vi "Traction Receipe Run Trial.vi"() -> ()   [LabVIEW 2025]
uses:
  Traction Receipe Enum.ctl
panel:
  out "SET entrainment Velocity":dbl
  out "Test Array Size":i32
  in  "SRR INDEX [ STRIBECK]":i32
  out "Stribeck Size":i32
  out "SET SRR":dbl
  out "Enum - READ":T1
  out "ELAPSED TIMER":dbl
  in  "START":bool
  out "BALL SET RPM":dbl
  out "DISC SET RPM":dbl
  in  "LOAD READ":dbl
  out "SET LOAD":dbl
  in  "TEMPERATURE READ":dbl
  out "SET TEMPERATURE":dbl
  out "Traction Size":i32
  out "DISC SPEED (rpm)":dbl=100.0 min=0.1 max=3000.0 step=0.1 format="%.1f"
  out "BALL SPEED (rpm)":dbl=100.0 min=0.1 max=3000.0 step=0.1 format="%.1f"
  in  "BALL WEAR TRACK":dbl=7.9
  in  "DISC WEARTRACK":dbl=16.0
  in  "SRR INDEX [ TRACTION]":i32
  in  "Start Index Type":i32
  in  "Enum - Menu":T1
  out "Ball (mm/sec)":dbl
  out "Disc (mm/sec)":dbl
  in  "Multicolumn Listbox":i32(listbox)
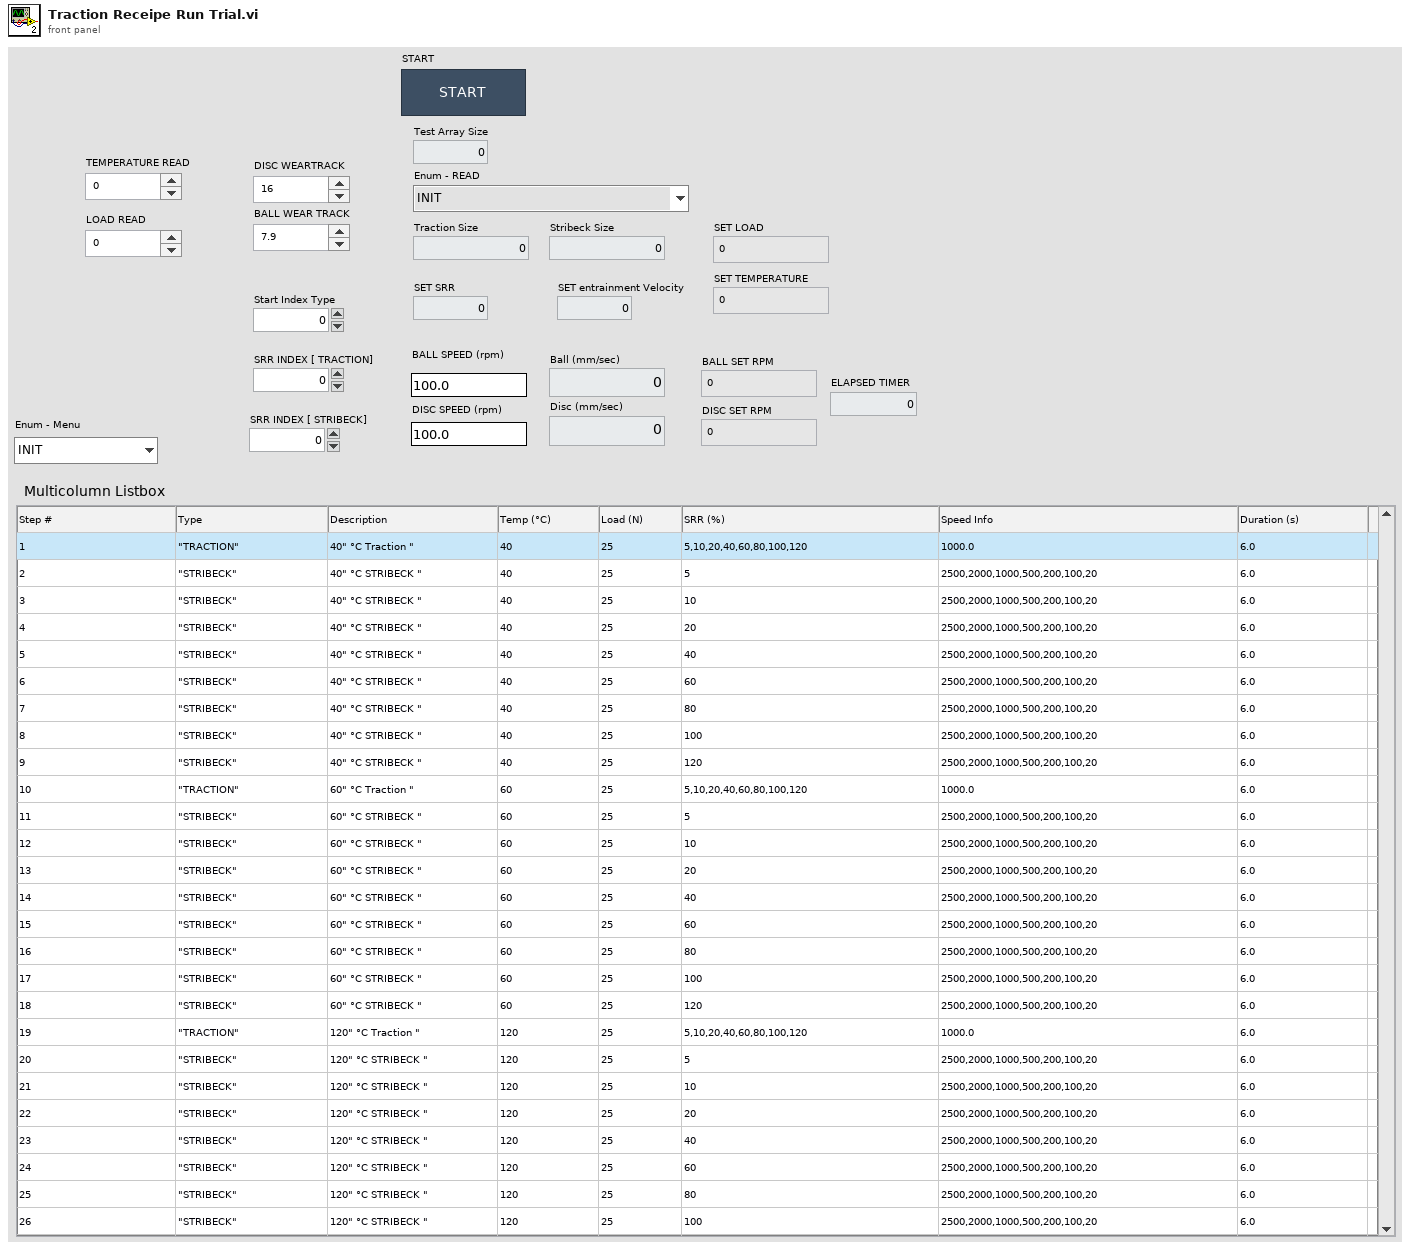
[diagram p1: front panel]
types:
  T1 = typedef "Traction Receipe Enum.ctl" = enum16{"INIT", "START", "TRACTION", "STRIBECK", "MAIN INDEX INCREMENT", "TEMPERATURE SET", "TEMPERATURE REACH", "CHURNING START", "CHURNING STOP", "LOAD", "LOAD REACHED", "SRR SET", "SRR WAIT", "SRR INCREMENT", "SPEED SET", "SPEED WAIT", "SPEED INCREMENT", "UNLOAD", "CLOSE"}
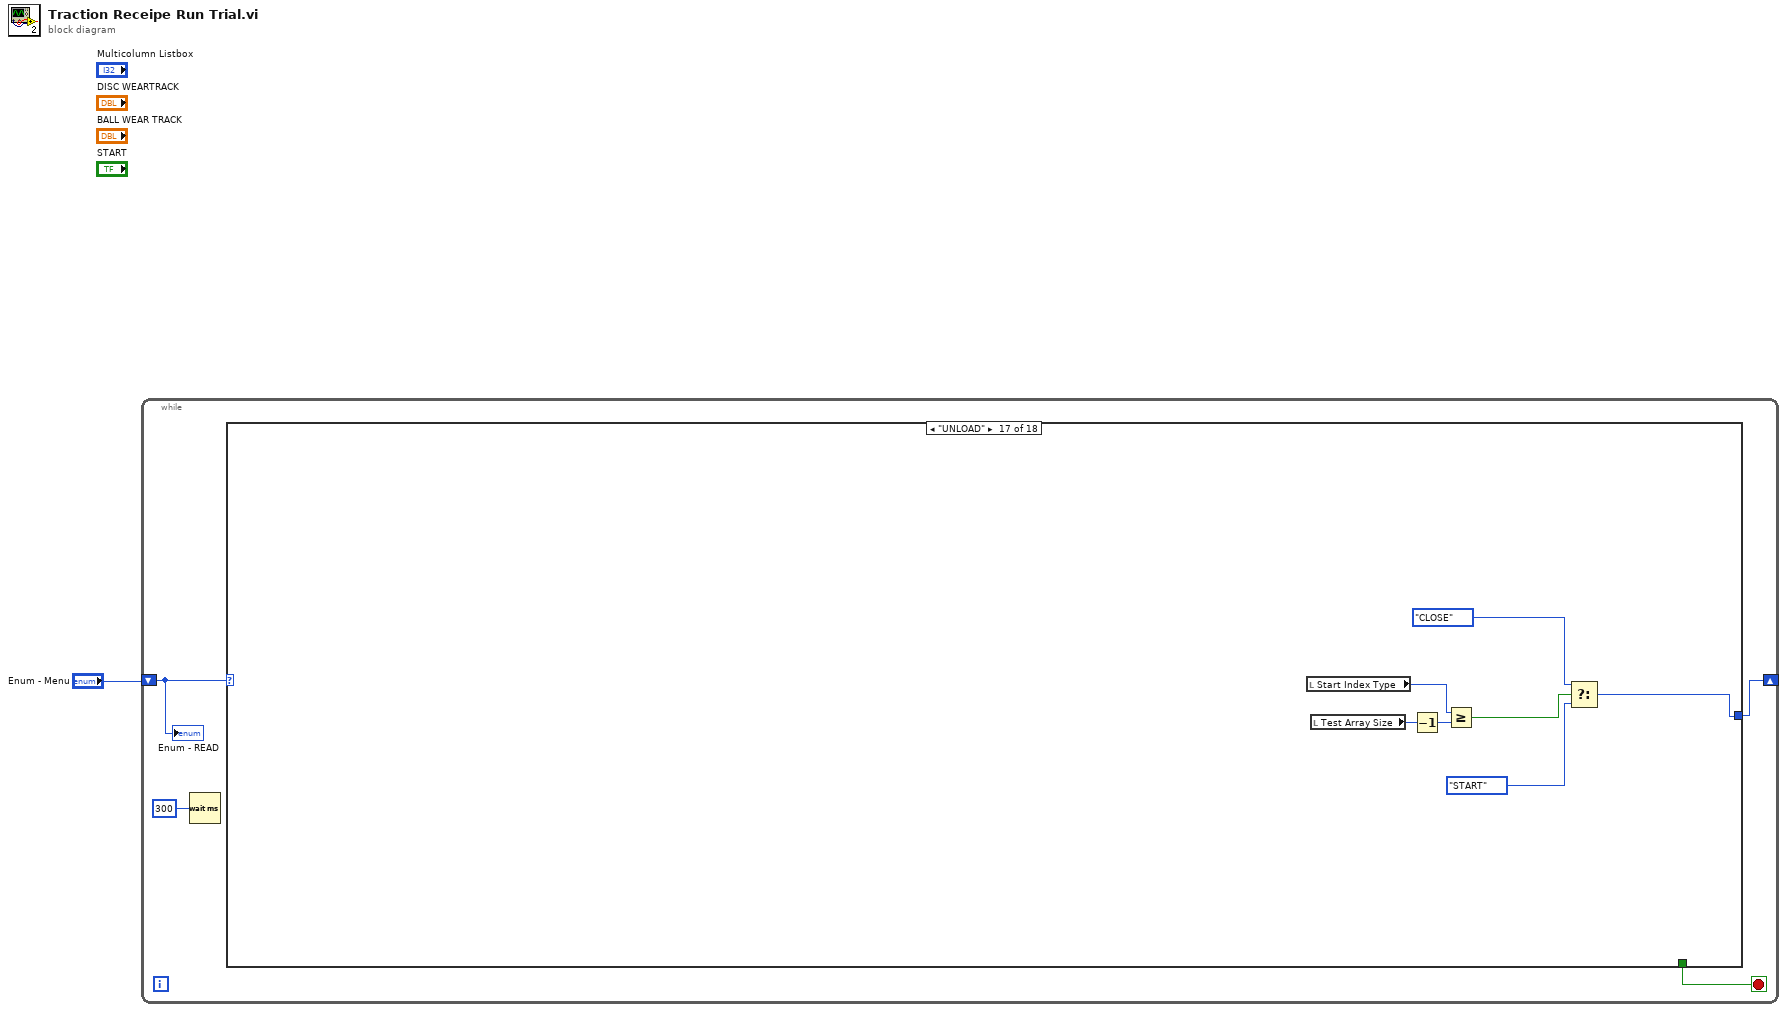
[diagram p0: block diagram]
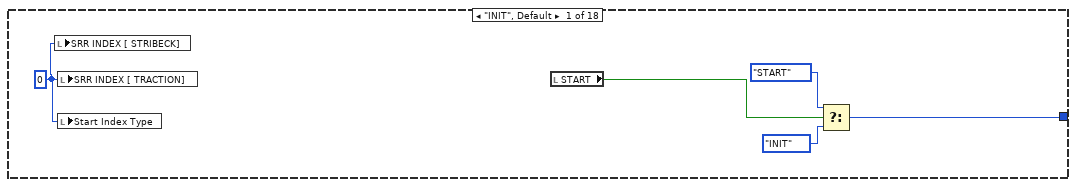
[diagram p2: hidden frame]
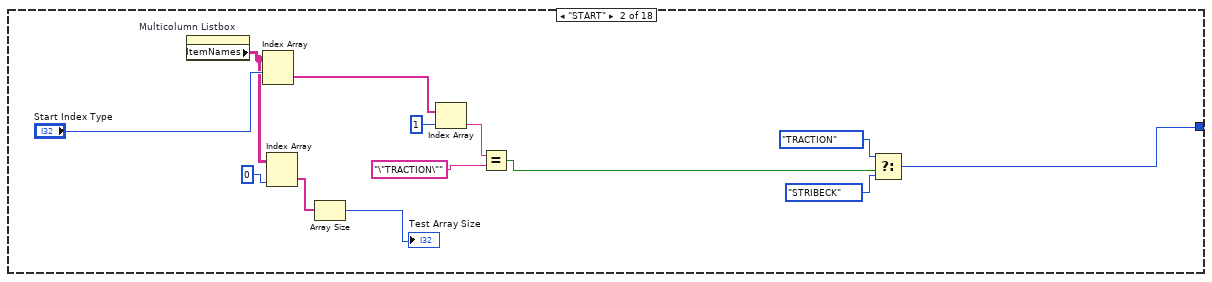
[diagram p3: hidden frame]
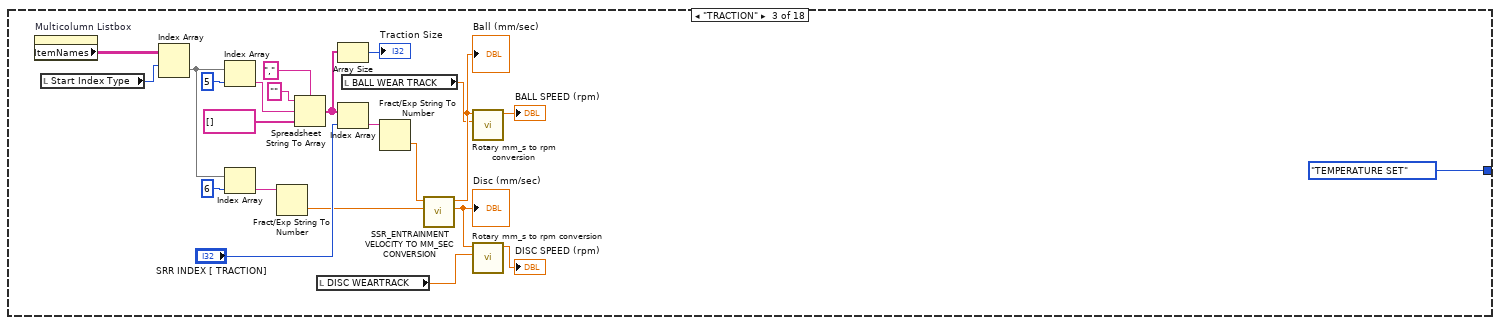
[diagram p4: hidden frame]
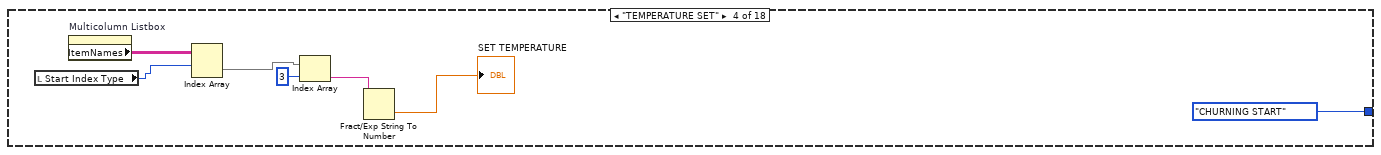
[diagram p5: hidden frame]
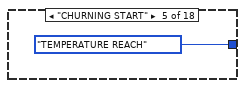
[diagram p6: hidden frame]
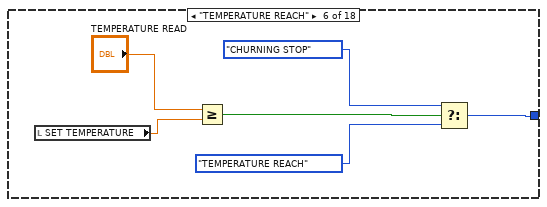
[diagram p7: hidden frame]
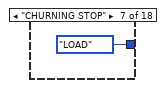
[diagram p8: hidden frame]
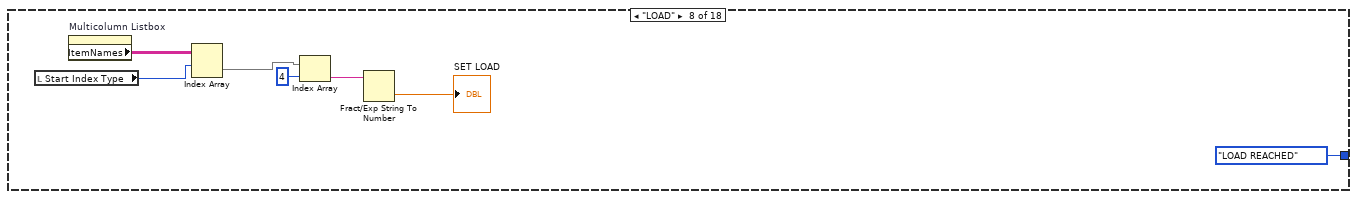
[diagram p9: hidden frame]
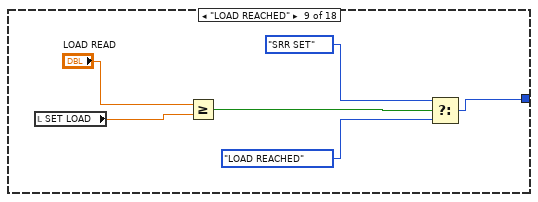
[diagram p10: hidden frame]
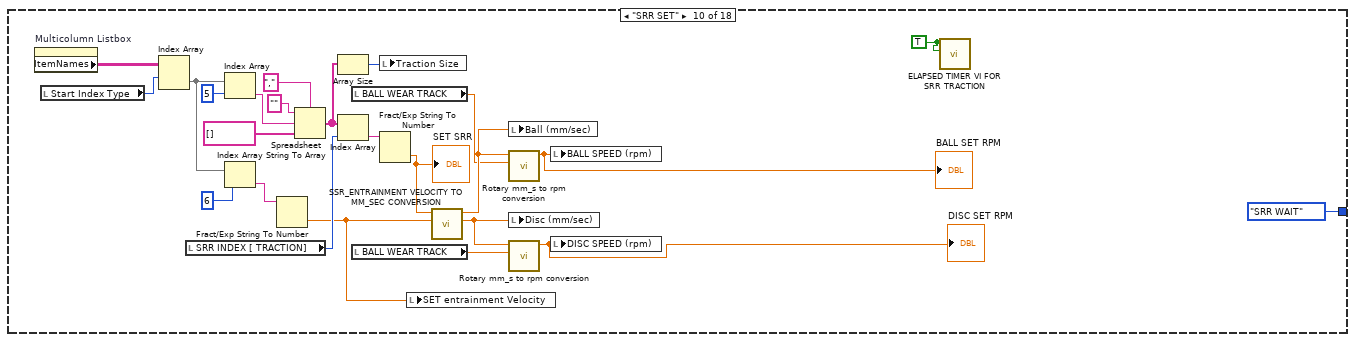
[diagram p11: hidden frame]
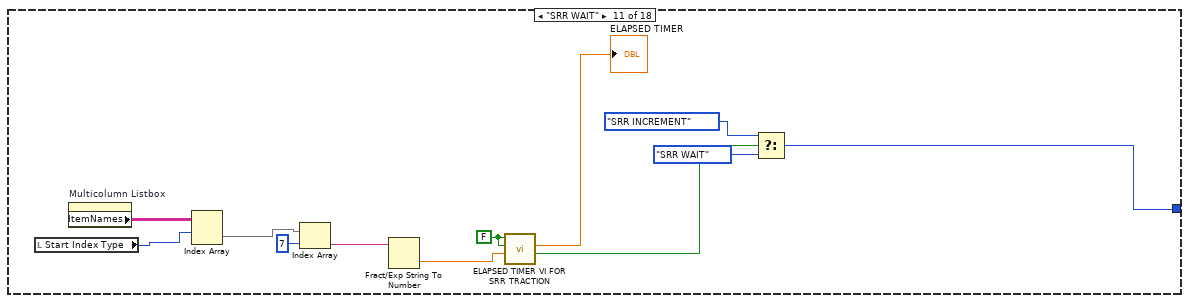
[diagram p12: hidden frame]
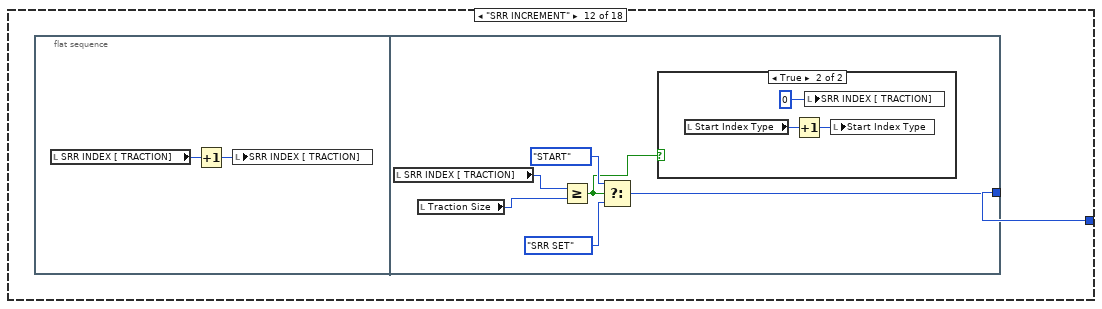
[diagram p13: hidden frame]
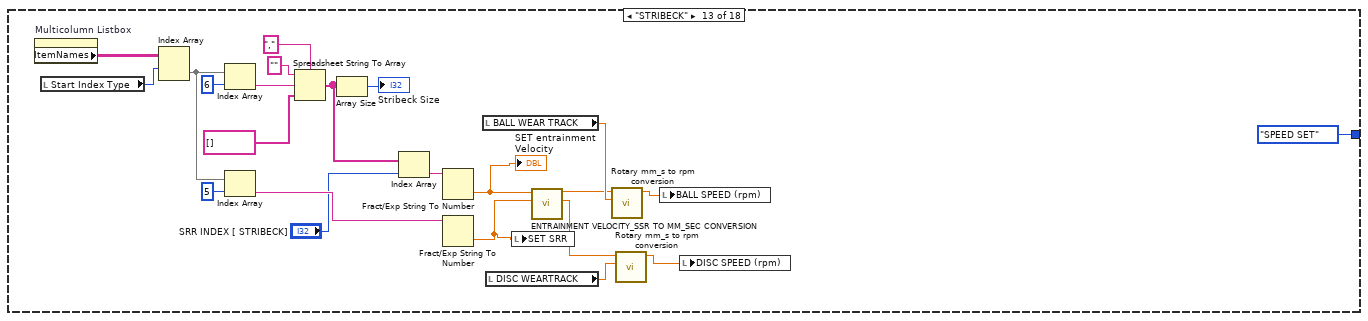
[diagram p15: hidden frame]
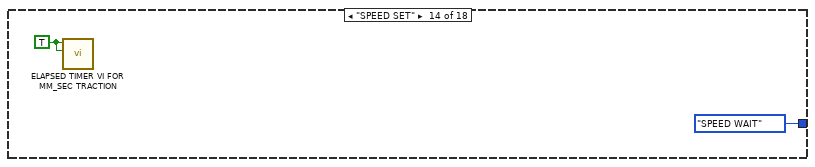
[diagram p16: hidden frame]
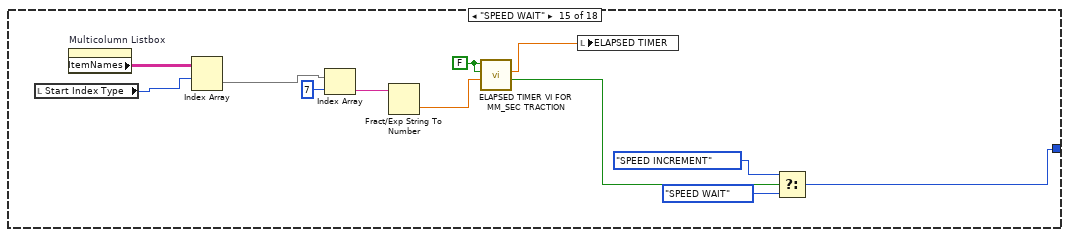
[diagram p17: hidden frame]
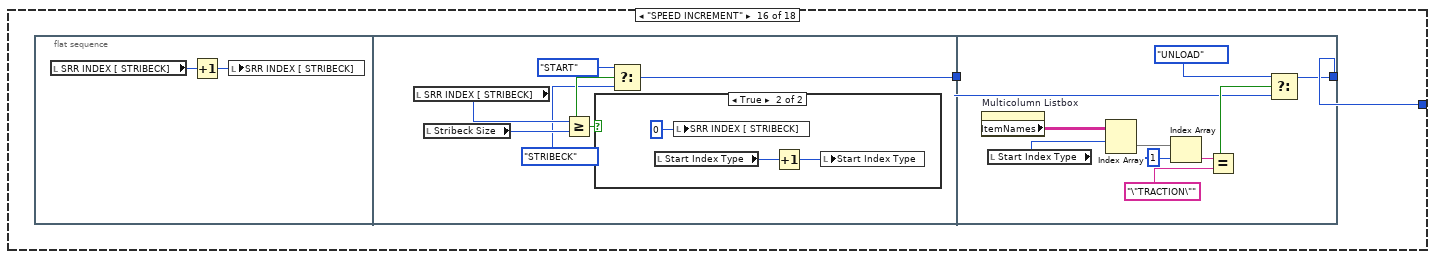
[diagram p18: hidden frame]
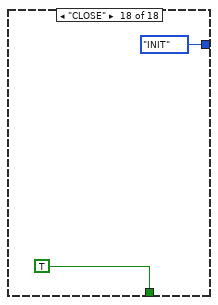
[diagram p20: hidden frame]
diagram:
  n1 = while {
    shift-right: [w4] -> _
    shift-left: "Enum - Menu" -> [w5]
    stop <- w3 stop-if-true
    n2 = Wait (ms)(milliseconds to wait=u32 300) -> ()  [unwired: 1 out]
    n3 = case shown="\"UNLOAD\"" w5 {
      tunnel: [w8 w15 Traction_Receipe_Enum."TEMPERATURE SET" ("Enum - Menu") Traction_Receipe_Enum."CHURNING START" ("Enum - Menu") Traction_Receipe_Enum."TEMPERATURE REACH" ("Enum - Menu") w55 Traction_Receipe_Enum."LOAD" ("Enum - Menu") Traction_Receipe_Enum."LOAD REACHED" ("Enum - Menu") w71 Traction_Receipe_Enum."SRR WAIT" ("Enum - Menu") w101 w111 Traction_Receipe_Enum."SPEED SET" ("Enum - Menu") Traction_Receipe_Enum."SPEED WAIT" ("Enum - Menu") w148 w161 w184 Traction_Receipe_Enum."INIT" ("Enum - Menu")] -> w4
      tunnel: [_ _ _ _ _ _ _ _ _ _ _ _ _ _ _ _ _ TRUE] -> w3
      frame "INIT", Default {
        w6 = 0 ("Start Index")
        n4 = local write "SRR INDEX [ STRIBECK]"(w6) -> ()
        n5 = local write "SRR INDEX [ TRACTION]"(w6) -> ()
        n6 = local write "Start Index Type"(w6) -> ()
        n7 = local read "START"() -> (w7:bool)
        n8 = Select(t=Traction_Receipe_Enum."START" ("Enum - Menu"), s=w7, f=Traction_Receipe_Enum."INIT" ("Enum - Menu")) -> (s? t:f=w8:T1)
      }
      frame "START" {
        n9 = property on="Multicolumn Listbox" class="MCListbox (strict)"() -> ("ItemNames"=w14:string[][])  [unwired: 2 in, 2 out]
        n10 = Index Array(array=w14, index (row)="Start Index Type") -> (element=w19:string[])  [unwired: 1 in]
        n11 = Index Array(array=w14, index (col)=0 ("index (row)")) -> (element=w13:string[])  [unwired: 1 in]
        n12 = Array Size(array=w13) -> (size(s)=→"Test Array Size":i32)
        n13 = Index Array(array=w19, index=1) -> (element=w21:string)
        n14 = Equal?(x=w21, y="\"TRACTION\"") -> (x = y?=w16:bool)
        n15 = Select(t=Traction_Receipe_Enum."TRACTION" ("Enum - Menu"), s=w16, f=Traction_Receipe_Enum."STRIBECK" ("Enum - Menu")) -> (s? t:f=w15:T1)
      }
      frame "TRACTION" {
        n16 = property on="Multicolumn Listbox" class="MCListbox (strict)"() -> ("ItemNames"=w41:string[][])  [unwired: 2 in, 2 out]
        n17 = local read "Start Index Type"() -> (w25:i32)
        n18 = Index Array(array=w41, index (row)=w25) -> (element=w40:string[])  [unwired: 1 in]
        n19 = Index Array(array=w40, index=5) -> (element=w39:string)
        n20 = Index Array(array=w40, index=6) -> (element=w34:string)
        n21 = Fract/Exp String To Number(string=w34) -> (number=w37:dbl)  [unwired: 3 in, 1 out]
        n22 = Spreadsheet String To Array(delimiter (Tab)=",", format string="", spreadsheet string=w39, array type (2D Dbl)=string[] []) -> (array=w28:string[])
        n23 = local read "DISC WEARTRACK"() -> (w24:dbl)
        n24 = Array Size(array=w28) -> (size(s)=→"Traction Size":i32)
        n25 = Index Array(array=w28, index="SRR INDEX [ TRACTION]") -> (element=w35:string)
        n26 = local read "BALL WEAR TRACK"() -> (w32:dbl)
        n27 = Fract/Exp String To Number(string=w35) -> (number=w36:dbl)  [unwired: 3 in, 1 out]
        n28 = call "SSR_ENTRAINMENT VELOCITY TO MM_SEC CONVERSION.vi"("Entrainment Speed"=w37, "Initial SSR"=w36) -> ("Disc"=w31:dbl, "Ball"=w33:dbl)  [unwired: 7 in, 1 out]
        "Disc (mm/sec)" <- w31
        "Ball (mm/sec)" <- w33
        n29 = call "Rotary mm_s to rpm conversion.vi"("Wear Track Diameter"=w32, "Enter initial Velocity (m/s)  3"=w33) -> ("Initial Speed (RPM) 2"=→"BALL SPEED (rpm)":dbl)  [unwired: 7 in, 2 out]
        n30 = call "Rotary mm_s to rpm conversion.vi"("Wear Track Diameter"=w24, "Enter initial Velocity (m/s)  3"=w31) -> ("Initial Speed (RPM) 2"=→"DISC SPEED (rpm)":dbl)  [unwired: 7 in, 2 out]
      }
      frame "TEMPERATURE SET" {
        n31 = local read "Start Index Type"() -> (w47:i32)
        n32 = property on="Multicolumn Listbox" class="MCListbox (strict)"() -> ("ItemNames"=w51:string[][])  [unwired: 2 in, 2 out]
        n33 = Index Array(array=w51, index (row)=w47) -> (element=w52:string[])  [unwired: 1 in]
        n34 = Index Array(array=w52, index=3) -> (element=w49:string)
        n35 = Fract/Exp String To Number(string=w49) -> (number=→"SET TEMPERATURE":dbl)  [unwired: 3 in, 1 out]
      }
      frame "CHURNING START" {
      }
      frame "TEMPERATURE REACH" {
        n36 = local read "SET TEMPERATURE"() -> (w59:dbl)
        n37 = Greater Or Equal?(x="TEMPERATURE READ", y=w59) -> (x >= y?=w58:bool)
        n38 = Select(t=Traction_Receipe_Enum."CHURNING STOP" ("Enum - Menu"), s=w58, f=Traction_Receipe_Enum."TEMPERATURE REACH" ("Enum - Menu")) -> (s? t:f=w55:T1)
      }
      frame "CHURNING STOP" {
      }
      frame "LOAD" {
        n39 = local read "Start Index Type"() -> (w62:i32)
        n40 = property on="Multicolumn Listbox" class="MCListbox (strict)"() -> ("ItemNames"=w67:string[][])  [unwired: 2 in, 2 out]
        n41 = Index Array(array=w67, index (row)=w62) -> (element=w68:string[])  [unwired: 1 in]
        n42 = Index Array(array=w68, index=4) -> (element=w66:string)
        n43 = Fract/Exp String To Number(string=w66) -> (number=→"SET LOAD":dbl)  [unwired: 3 in, 1 out]
      }
      frame "LOAD REACHED" {
        n44 = local read "SET LOAD"() -> (w69:dbl)
        n45 = Greater Or Equal?(x="LOAD READ", y=w69) -> (x >= y?=w74:bool)
        n46 = Select(t=Traction_Receipe_Enum."SRR SET" ("Enum - Menu"), s=w74, f=Traction_Receipe_Enum."LOAD REACHED" ("Enum - Menu")) -> (s? t:f=w71:T1)
      }
      frame "SRR SET" {
        w97 = TRUE ("PAUSE")
        n47 = property on="Multicolumn Listbox" class="MCListbox (strict)"() -> ("ItemNames"=w92:string[][])  [unwired: 2 in, 2 out]
        n48 = local read "Start Index Type"() -> (w83:i32)
        n49 = Index Array(array=w92, index (row)=w83) -> (element=w91:string[])  [unwired: 1 in]
        n50 = local read "SRR INDEX [ TRACTION]"() -> (w95:i32)
        n51 = Index Array(array=w91, index=5) -> (element=w90:string)
        n52 = Index Array(array=w91, index=6) -> (element=w87:string)
        n53 = Fract/Exp String To Number(string=w87) -> (number=w75:dbl)  [unwired: 3 in, 1 out]
        n54 = Spreadsheet String To Array(delimiter (Tab)=",", format string="", spreadsheet string=w90, array type (2D Dbl)=string[] []) -> (array=w84:string[])
        n55 = Array Size(array=w84) -> (size(s)=w96:i32)
        n56 = Index Array(array=w84, index=w95) -> (element=w88:string)
        n57 = local read "BALL WEAR TRACK"() -> (w86:dbl)
        n58 = local read "BALL WEAR TRACK"() -> (w85:dbl)
        n59 = local write "Traction Size"(w96) -> ()
        n60 = Fract/Exp String To Number(string=w88) -> (number=w89:dbl)  [unwired: 3 in, 1 out]
        "SET SRR" <- w89
        n61 = local write "SET entrainment Velocity"(w75) -> ()
        n62 = call "SSR_ENTRAINMENT VELOCITY TO MM_SEC CONVERSION.vi"("Entrainment Speed"=w75, "Initial SSR"=w89) -> ("Disc"=w94:dbl, "Ball"=w93:dbl)  [unwired: 7 in, 1 out]
        n63 = local write "Ball (mm/sec)"(w93) -> ()
        n64 = call "Rotary mm_s to rpm conversion.vi"("Wear Track Diameter"=w86, "Enter initial Velocity (m/s)  3"=w93) -> ("Initial Speed (RPM) 2"=w77:dbl)  [unwired: 7 in, 2 out]
        "BALL SET RPM" <- w77
        n65 = local write "Disc (mm/sec)"(w94) -> ()
        n66 = call "Rotary mm_s to rpm conversion.vi"("Wear Track Diameter"=w85, "Enter initial Velocity (m/s)  3"=w94) -> ("Initial Speed (RPM) 2"=w76:dbl)  [unwired: 7 in, 2 out]
        "DISC SET RPM" <- w76
        n67 = local write "BALL SPEED (rpm)"(w77) -> ()
        n68 = local write "DISC SPEED (rpm)"(w76) -> ()
        n69 = call "ELAPSED TIMER VI FOR SRR TRACTION.vi"("RESET"=w97, "PAUSE"=w97) -> ()  [unwired: 7 in, 3 out]
      }
      frame "SRR WAIT" {
        w106 = FALSE ("PAUSE")
        n70 = local read "Start Index Type"() -> (w99:i32)
        n71 = property on="Multicolumn Listbox" class="MCListbox (strict)"() -> ("ItemNames"=w109:string[][])  [unwired: 2 in, 2 out]
        n72 = Index Array(array=w109, index (row)=w99) -> (element=w110:string[])  [unwired: 1 in]
        n73 = Index Array(array=w110, index=7) -> (element=w108:string)
        n74 = Fract/Exp String To Number(string=w108) -> (number=w105:dbl)  [unwired: 3 in, 1 out]
        n75 = call "ELAPSED TIMER VI FOR SRR TRACTION.vi"("TARGET"=w105, "RESET"=w106, "PAUSE"=w106) -> ("ELAPSED INDICATION"=w104:bool, "ELAPSED TIMER"=→"ELAPSED TIMER":dbl)  [unwired: 6 in, 1 out]
        n76 = Select(t=Traction_Receipe_Enum."SRR INCREMENT" ("Enum - Menu"), s=w104, f=Traction_Receipe_Enum."SRR WAIT") -> (s? t:f=w101:T1)
      }
      frame "SRR INCREMENT" {
        n77 = flat-sequence {
          tunnel: [w116] -> w111
          frame #0 {
            n78 = local read "SRR INDEX [ TRACTION]"() -> (w113:i32)
            n79 = Increment(x=w113) -> (x+1=w112:i32)
            n80 = local write "SRR INDEX [ TRACTION]"(w112) -> ()
          }
          frame #1 {
            n81 = local read "SRR INDEX [ TRACTION]"() -> (w114:i32)
            n82 = local read "Traction Size"() -> (w119:i32)
            n83 = Greater Or Equal?(x=w114, y=w119) -> (x >= y?=w115:bool)
            n84 = Select(t=Traction_Receipe_Enum."START" ("Enum - Menu"), s=w115, f=Traction_Receipe_Enum."SRR SET" ("Enum - Menu")) -> (s? t:f=w116:T1)
            n85 = case shown="True" w115 {
              frame False {
              }
              frame True {
                n86 = local read "Start Index Type"() -> (w122:i32)
                n87 = Increment(x=w122) -> (x+1=w121:i32)
                n88 = local write "SRR INDEX [ TRACTION]"(0 ("SRR INDEX [ TRACTION]")) -> ()
                n89 = local write "Start Index Type"(w121) -> ()
              }
            }
          }
        }
      }
      frame "STRIBECK" {
        n90 = property on="Multicolumn Listbox" class="MCListbox (strict)"() -> ("ItemNames"=w130:string[][])  [unwired: 2 in, 2 out]
        n91 = local read "Start Index Type"() -> (w131:i32)
        n92 = Index Array(array=w130, index (row)=w131) -> (element=w134:string[])  [unwired: 1 in]
        n93 = Index Array(array=w134, index=6) -> (element=w132:string)
        n94 = Index Array(array=w134, index=5) -> (element=w138:string)
        n95 = Spreadsheet String To Array(delimiter (Tab)=",", format string="", spreadsheet string=w132, array type (2D Dbl)=string[] []) -> (array=w136:string[])
        n96 = Array Size(array=w136) -> (size(s)=→"Stribeck Size":i32)
        n97 = Index Array(array=w136, index="SRR INDEX [ STRIBECK]") -> (element=w137:string)
        n98 = Fract/Exp String To Number(string=w137) -> (number=w124:dbl)  [unwired: 3 in, 1 out]
        "SET entrainment Velocity" <- w124
        n99 = Fract/Exp String To Number(string=w138) -> (number=w123:dbl)  [unwired: 3 in, 1 out]
        n100 = local read "BALL WEAR TRACK"() -> (w140:dbl)
        n101 = local read "DISC WEARTRACK"() -> (w142:dbl)
        n102 = local write "SET SRR"(w123) -> ()
        n103 = call "ENTRAINMENT VELOCITY_SSR TO MM_SEC CONVERSION.vi"("SSR"=w123, "INITIAL Entrainment Speed"=w124) -> ("Disc"=w141:dbl, "Ball"=w139:dbl)  [unwired: 7 in, 1 out]
        n104 = call "Rotary mm_s to rpm conversion.vi"("Wear Track Diameter"=w140, "Enter initial Velocity (m/s)  3"=w139) -> ("Initial Speed (RPM) 2"=w143:dbl)  [unwired: 7 in, 2 out]
        n105 = call "Rotary mm_s to rpm conversion.vi"("Wear Track Diameter"=w142, "Enter initial Velocity (m/s)  3"=w141) -> ("Initial Speed (RPM) 2"=w144:dbl)  [unwired: 7 in, 2 out]
        n106 = local write "BALL SPEED (rpm)"(w143) -> ()
        n107 = local write "DISC SPEED (rpm)"(w144) -> ()
      }
      frame "SPEED SET" {
        w146 = TRUE ("PAUSE")
        n108 = call "ELAPSED TIMER VI FOR MM_SEC TRACTION.vi"("RESET"=w146, "PAUSE"=w146) -> ()  [unwired: 7 in, 3 out]
      }
      frame "SPEED WAIT" {
        w153 = FALSE ("PAUSE")
        n109 = local read "Start Index Type"() -> (w156:i32)
        n110 = property on="Multicolumn Listbox" class="MCListbox (strict)"() -> ("ItemNames"=w158:string[][])  [unwired: 2 in, 2 out]
        n111 = Index Array(array=w158, index (row)=w156) -> (element=w159:string[])  [unwired: 1 in]
        n112 = Index Array(array=w159, index=7) -> (element=w157:string)
        n113 = Fract/Exp String To Number(string=w157) -> (number=w154:dbl)  [unwired: 3 in, 1 out]
        n114 = call "ELAPSED TIMER VI FOR MM_SEC TRACTION.vi"("TARGET"=w154, "RESET"=w153, "PAUSE"=w153) -> ("ELAPSED INDICATION"=w149:bool, "ELAPSED TIMER"=w152:dbl)  [unwired: 6 in, 1 out]
        n115 = local write "ELAPSED TIMER"(w152) -> ()
        n116 = Select(t=Traction_Receipe_Enum."SPEED INCREMENT" ("Enum - Menu"), s=w149, f=Traction_Receipe_Enum."SPEED WAIT") -> (s? t:f=w148:T1)
      }
      frame "SPEED INCREMENT" {
        n117 = flat-sequence {
          tunnel: [w164] -> w160
          tunnel: [w176] -> w161
          tunnel: w160 -> [w174]
          frame #0 {
            n118 = local read "SRR INDEX [ STRIBECK]"() -> (w163:i32)
            n119 = Increment(x=w163) -> (x+1=w162:i32)
            n120 = local write "SRR INDEX [ STRIBECK]"(w162) -> ()
          }
          frame #1 {
            n121 = local read "SRR INDEX [ STRIBECK]"() -> (w168:i32)
            n122 = local read "Stribeck Size"() -> (w169:i32)
            n123 = Greater Or Equal?(x=w168, y=w169) -> (x >= y?=w166:bool)
            n124 = case shown="True" w166 {
              frame False {
              }
              frame True {
                n125 = local read "Start Index Type"() -> (w172:i32)
                n126 = local write "SRR INDEX [ STRIBECK]"(0 ("SRR INDEX [ STRIBECK]")) -> ()
                n127 = Increment(x=w172) -> (x+1=w171:i32)
                n128 = local write "Start Index Type"(w171) -> ()
              }
            }
            n129 = Select(t=Traction_Receipe_Enum."START" ("Enum - Menu"), s=w166, f=Traction_Receipe_Enum."STRIBECK") -> (s? t:f=w164:T1)
          }
          frame #2 {
            n130 = property on="Multicolumn Listbox" class="MCListbox (strict)"() -> ("ItemNames"=w181:string[][])  [unwired: 2 in, 2 out]
            n131 = local read "Start Index Type"() -> (w182:i32)
            n132 = Index Array(array=w181, index (row)=w182) -> (element=w179:string[])  [unwired: 1 in]
            n133 = Index Array(array=w179, index=1) -> (element=w180:string)
            n134 = Equal?(x=w180, y="\"TRACTION\"") -> (x = y?=w175:bool)
            n135 = Select(t=Traction_Receipe_Enum."UNLOAD", s=w175, f=w174) -> (s? t:f=w176:T1)
          }
        }
      }
      frame "UNLOAD" {
        n136 = local read "Start Index Type"() -> (w188:i32)
        n137 = local read "Test Array Size"() -> (w189:i32)
        n138 = Decrement(x=w189) -> (x-1=w183:i32)
        n139 = Greater Or Equal?(x=w188, y=w183) -> (x >= y?=w187:bool)
        n140 = Select(t=Traction_Receipe_Enum."CLOSE" ("Enum - Menu"), s=w187, f=Traction_Receipe_Enum."START" ("Enum - Menu")) -> (s? t:f=w184:T1)
      }
      frame "CLOSE" {
      }
    }
    "Enum - READ" <- w5
  }
